vi "no index.vi"() -> ()   [LabVIEW 2020]
panel:
  out "Data In":u8[](array[numeric]) format="%.0x"
  out "6":u64 format="%.0x"
  out "5":u64 format="%.0x"
  out "4":u64 format="%.0x"
  out "3":u64 format="%.0x"
  out "2":u64 format="%.0x"
  out "1":u64 format="%.0x"
  out "Batch Length":i32
  out "Actual Bitrate kHz 2":i32=1000
  in  "SDI":u64[](array[numeric]) format="%.0x"
  out "dup Cheetah Handle":i32
  out "Total Shifted Out":i32
  out "Actual Bitrate kHz":i32=1000
  out "error out":errorcluster
  in  "Rds per Sec":dbl=2000.0 max=2000000000.0
  in  "SCLK (kHz)":i32=2000 min=0
  out "Cheetah Handle":i32
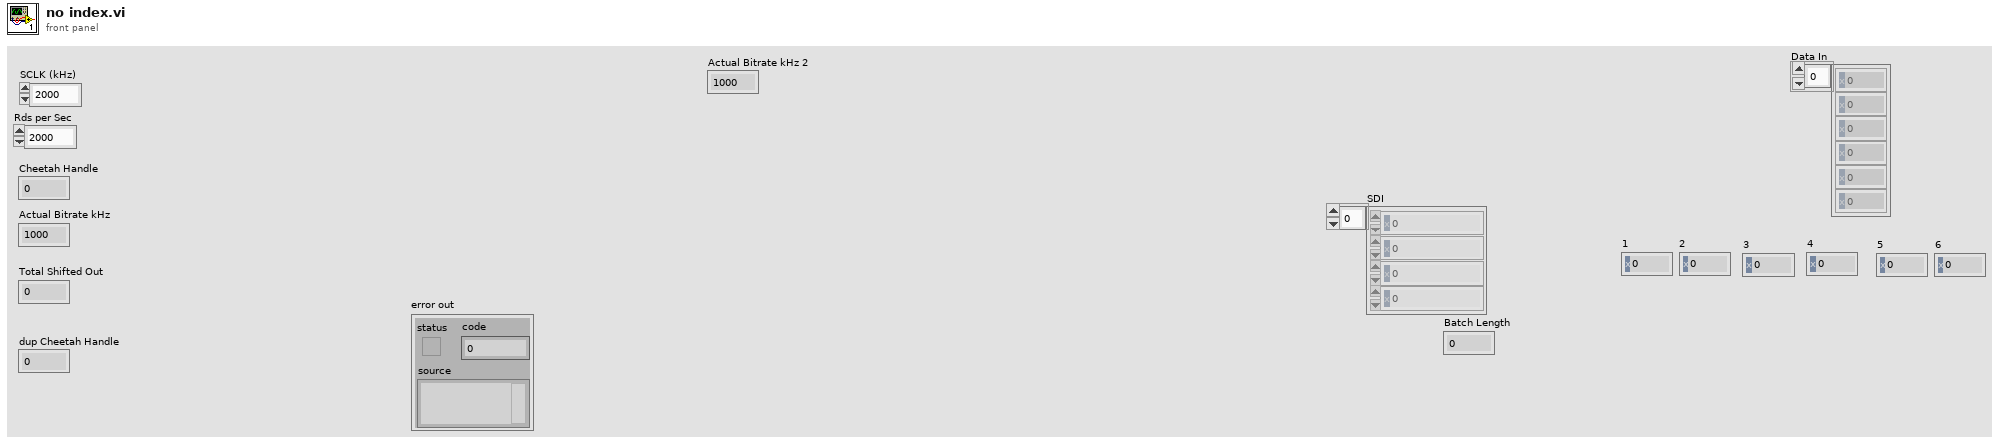
[diagram p1: front panel]
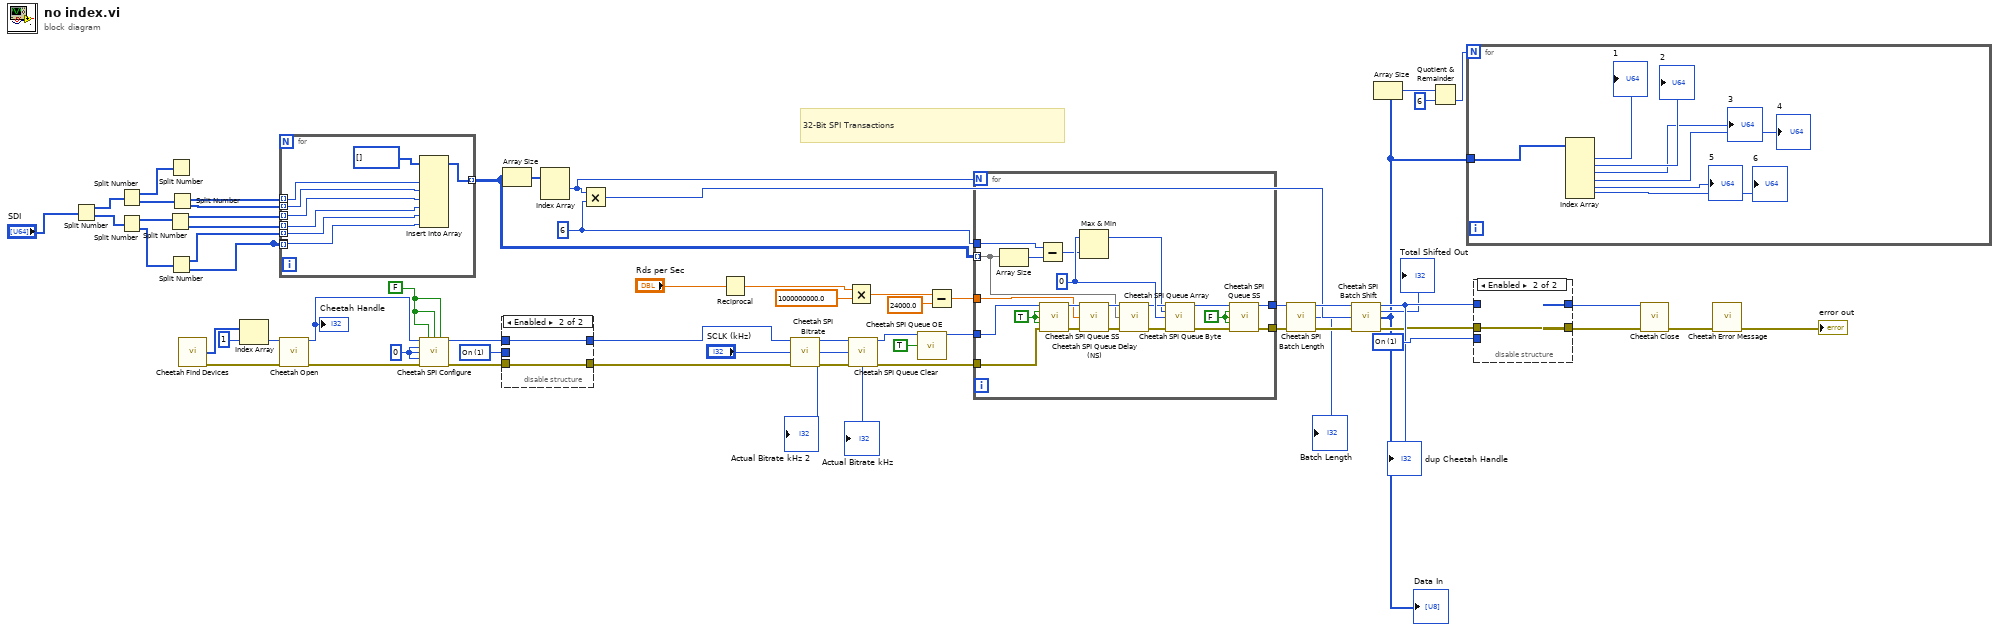
[diagram p0: block diagram]
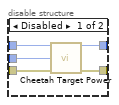
[diagram p2: hidden frame]
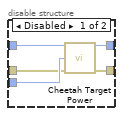
[diagram p3: hidden frame]
diagram:
  w18 = 6 ("y")
  w42 = u16 1 items=["Off", "On", "Query"] ("Requested Configuration (2: Query)")
  w43 = u16 1 items=["Off", "On", "Query"] ("Requested Configuration (2: Query)")
  w58 = FALSE
  w60 = 0
  # "32-Bit SPI Transactions"
  n1 = Split Number(x="SDI") -> (hi(x)=w29:u32[], lo(x)=w28:u32[])
  n2 = Split Number(x=w29) -> (hi(x)=w5:u16[], lo(x)=w4:u16[])
  n3 = Split Number(x=w28) -> (hi(x)=w8:u16[], lo(x)=w7:u16[])
  n4 = Split Number(x=w8) -> (hi(x)=w12:u8[], lo(x)=w11:u8[])
  n5 = Split Number(x=w5) -> ()  [unwired: 2 out]
  n6 = Split Number(x=w7) -> (hi(x)=w10:u8[], lo(x)=w9:u8[])
  n7 = Split Number(x=w4) -> (hi(x)=w3:u8[], lo(x)=w2:u8[])
  n8 = call <instrlib>:"Cheetah Find Devices.vi"() -> ("Ports"=w61:u16[], "error out"=w57:errorcluster)  [unwired: 13 in, 1 out]
  n9 = Index Array(array=w61, index=1) -> (element=w49:u16)
  n10 = for {
    tunnel: w12 -> [w66] mode=indexing
    tunnel: [w70] -> w27 mode=indexing
    tunnel: w10 -> [w64] mode=indexing
    tunnel: w9 -> [w63] mode=indexing
    tunnel: w9 -> [_] mode=indexing
    tunnel: w11 -> [w65] mode=indexing
    tunnel: w3 -> [w68] mode=indexing
    tunnel: w2 -> [w67] mode=indexing
    n11 = Insert Into Array(array=u8[] [], new element #1=w68, new element #2=w67, new element #3=w66, new element #4=w65, new element #5=w64, new element #6=w63) -> (w70:u8[])  [unwired: 1 in]
  }
  n12 = call <instrlib>:"Cheetah Open.vi"("Port Number (0)"=w49, "error in (no error)"=w57) -> ("Cheetah Handle"=w54:i32, "error out"=w56:errorcluster)  [unwired: 12 in]
  "Cheetah Handle" <- w54
  n13 = call <instrlib>:"Cheetah SPI Configure.vi"("Cheetah Handle"=w54, "SS0 Active High? (False)"=w58, "SS1 Active High? (False)"=w58, "SS2 Active High? (False)"=w58, "Polarity (0: Rising/Falling)"=w60, "Phase (0: Sample/Setup)"=w60, "Bitorder (0: MSB)"=w60, "error in (no error)"=w56) -> ("dup Cheetah Handle"=w53:i32, "error out"=w55:errorcluster)  [unwired: 6 in]
  n14 = disable-structure shown="Enabled" {
    disable-tunnel: w55 -> [w75 w76]
    disable-tunnel: w53 -> [w74 w77]
    disable-tunnel: [w73 w76] -> w52
    disable-tunnel: [w72 w77] -> w50
    disable-tunnel: w42 -> [w71 _]
    frame Disabled {
      n15 = call <instrlib>:"Cheetah Target Power.vi"("Cheetah Handle"=w74, "Requested Configuration (2: Query)"=w71, "error in (no error)"=w75) -> ("dup Cheetah Handle"=w72:i32, "error out"=w73:errorcluster)  [unwired: 10 in, 1 out]
    }
    frame Enabled {
    }
  }
  n16 = Array Size(array=w27) -> (size(s)=w41:i32[])
  n17 = Index Array(array=w41) -> (element #1=w14:i32)  [unwired: 2 in, 1 out]
  n18 = Multiply(x=w14, y=w18) -> (x*y=w13:i32)
  n19 = Reciprocal(x="Rds per Sec") -> (1/x=w20:dbl)
  n20 = call <instrlib>:"Cheetah SPI Bitrate.vi"("Cheetah Handle"=w50, "Requested Bitrate kHz (1000)"="SCLK (kHz)", "error in (no error)"=w52) -> ("dup Cheetah Handle"=w48:i32, "Actual Bitrate kHz"=→"Actual Bitrate kHz" →"Actual Bitrate kHz 2":i32, "error out"=w47:errorcluster)  [unwired: 10 in]
  n21 = Multiply(x=w20, y=1000000000.0) -> (x*y=w23:dbl)
  n22 = call <instrlib>:"Cheetah SPI Queue Clear.vi"("Cheetah Handle"=w48, "error in (no error)"=w47) -> ("dup Cheetah Handle"=w40:i32, "error out"=w59:errorcluster)  [unwired: 12 in]
  n23 = call <instrlib>:"Cheetah SPI Queue OE.vi"("Cheetah Handle"=w40, "Output Enable (on)"=TRUE) -> ("dup Cheetah Handle"=w39:i32)  [unwired: 12 in, 1 out]
  n24 = Subtract(x=w23, y=24000.0) -> (x-y=w21:dbl)
  n25 = for {
    N: w14 -> [_]
    tunnel: w59 -> [w84]
    tunnel: w39 -> [w85]
    tunnel: w27 -> [w86] mode=indexing
    tunnel: [w83] -> w37
    tunnel: [w82] -> w36
    tunnel: w21 -> [w79]
    tunnel: w18 -> [w80]
    w90 = FALSE
    w93 = 0
    w81 = TRUE
    n26 = Array Size(array=w86) -> (size(s)=w87:i32)
    n27 = Subtract(x=w80, y=w87) -> (x-y=w91:i32)
    n28 = call <instrlib>:"Cheetah SPI Queue SS.vi"("Cheetah Handle"=w85, "SS0 Assert? (True)"=w81, "SS1 Assert? (True)"=w81, "SS2 Assert? (True)"=w81, "error in (no error)"=w84) -> ("dup Cheetah Handle"=w98:i32, "error out"=w97:errorcluster)  [unwired: 9 in]
    n29 = Max & Min(x=w93, y=w91) -> (max(x,y)=w78:i32)  [unwired: 1 out]
    n30 = call <instrlib>:"Cheetah SPI Queue Delay (NS).vi"("Cheetah Handle"=w98, "Delay NS (1000)"=w79, "error in (no error)"=w97) -> ("dup Cheetah Handle"=w96:i32, "error out"=w95:errorcluster)  [unwired: 10 in, 1 out]
    n31 = call <instrlib>:"Cheetah SPI Queue Array.vi"("Cheetah Handle"=w96, "Data Out (none)"=w86, "error in (no error)"=w95) -> ("dup Cheetah Handle"=w92:i32, "error out"=w94:errorcluster)  [unwired: 11 in]
    n32 = call <instrlib>:"Cheetah SPI Queue Byte.vi"("Cheetah Handle"=w92, "Byte Count (1)"=w78, "Byte Value (0x00)"=w93, "error in (no error)"=w94) -> ("dup Cheetah Handle"=w89:i32, "error out"=w88:errorcluster)  [unwired: 10 in]
    n33 = call <instrlib>:"Cheetah SPI Queue SS.vi"("Cheetah Handle"=w89, "SS0 Assert? (True)"=w90, "SS1 Assert? (True)"=w90, "SS2 Assert? (True)"=w90, "error in (no error)"=w88) -> ("dup Cheetah Handle"=w82:i32, "error out"=w83:errorcluster)  [unwired: 9 in]
  }
  n34 = call <instrlib>:"Cheetah SPI Batch Length.vi"("Cheetah Handle"=w36, "error in (no error)"=w37) -> ("dup Cheetah Handle"=w35:i32, "Batch Length"=→"Batch Length":i32, "error out"=w34:errorcluster)  [unwired: 11 in]
  n35 = call <instrlib>:"Cheetah SPI Batch Shift.vi"("Cheetah Handle"=w35, "Max Bytes to Retrieve (256)"=w13, "error in (no error)"=w34) -> ("dup Cheetah Handle"=w33:i32, "Total Shifted Out"=→"Total Shifted Out":i32, "Data In"=w15:u8[], "error out"=w26:errorcluster)  [unwired: 9 in]
  "dup Cheetah Handle" <- w33
  "Data In" <- w15
  n36 = Array Size(array=w15) -> (size(s)=w32:i32)
  n37 = Quotient & Remainder(x=w32, y=6) -> (floor(x/y)=w30:i32)  [unwired: 1 out]
  n38 = for {
    N: w30 -> [_]
    tunnel: w15 -> [w105]
    n39 = Index Array(array=w105) -> (element #1=→"1":u8, element #2=→"2":u8, element #3=→"3":u8, element #4=→"4":u8, element #5=→"5":u8, element #6=→"6":u8)  [unwired: 6 in]
  }
  n40 = disable-structure shown="Enabled" {
    disable-tunnel: [w110 _] -> w46
    disable-tunnel: [w109 w111] -> w45
    disable-tunnel: w43 -> [w108 _]
    disable-tunnel: w33 -> [w107 _]
    disable-tunnel: w26 -> [w106 w111]
    frame Disabled {
      n41 = call <instrlib>:"Cheetah Target Power.vi"("Cheetah Handle"=w107, "Requested Configuration (2: Query)"=w108, "error in (no error)"=w106) -> ("dup Cheetah Handle"=w110:i32, "error out"=w109:errorcluster)  [unwired: 10 in, 1 out]
    }
    frame Enabled {
    }
  }
  n42 = call <instrlib>:"Cheetah Close.vi"("Cheetah Handle"=w46, "error in (no error)"=w45) -> ("error out"=w44:errorcluster)  [unwired: 12 in, 1 out]
  n43 = call <instrlib>:"Cheetah Error Message.vi"("error in (no error)"=w44) -> ("error out"=→"error out":errorcluster)  [unwired: 10 in, 4 out]
